vi "VI-Center XControl Property FP Value.vi"(0 "VI in":refnum<vi>, 2 "Data Type In":variant, 11 "error in (no error)":errorcluster) -> (4 "VI out":refnum<vi>, 15 "error out":errorcluster)   [LabVIEW 2015]
uses:
  <vilib>/Utility/traverseref.llb/TRef TravTarget.ctl
panel:
  in  "height":i16=200
  in  "width":i16=200
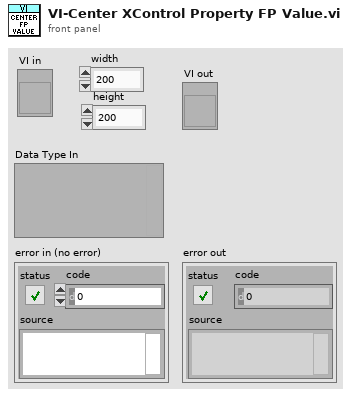
[diagram p1: front panel]
types:
  T1 = typedef "TRef TravTarget.ctl" = enum16{"FP", "BD", "Other"}
  T2 = typedef "LVRectTypeDef.ctl" = cluster{"Left":i16, "Top":i16, "Right":i16, "Bottom":i16}
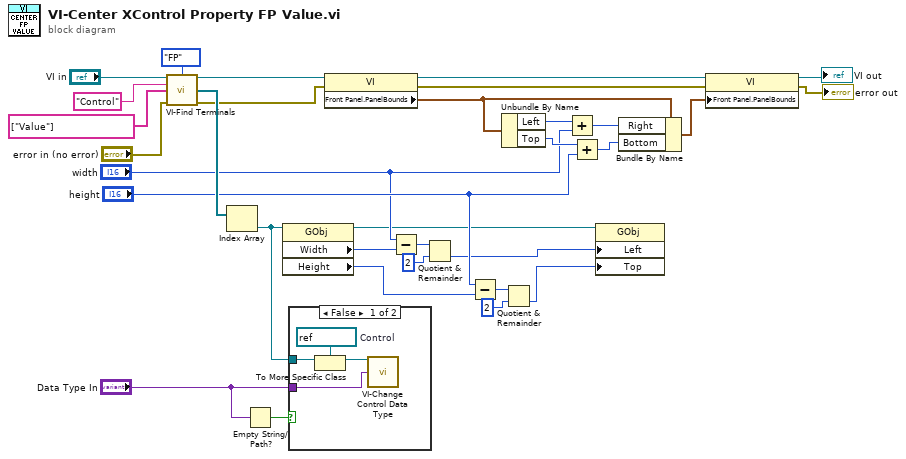
[diagram p0: block diagram]
diagram:
  n1 = call "VI-Find Terminals.vi"("VI in"="VI in", "Traverse Target"=TRef_TravTarget."FP", "Class Name"="Control", "Names"=string[] ["Value"], "error in (no error)"="error in (no error)") -> ("VI out"=w24:refnum<vi>, "Array"=w22:refnum<vi>[], "error out"=w17:errorcluster)  [unwired: 8 in]
  n2 = Index Array(array=w22) -> (element=w3:refnum<vi>)  [unwired: 1 in]
  n3 = Empty String/Path?(string/path="Data Type In") -> (empty?=w1:bool)
  n4 = property class="GObj"(reference=w3) -> (reference out=w5:refnum<vi>, "Width"=w6:u32, "Height"=w7:u32)  [unwired: 1 in, 1 out]
  n5 = case shown="False" w1 {
    tunnel: w3 -> [w34 _]
    tunnel: "Data Type In" -> [w33 _]
    frame False {
      w35 = refnum<vi> refnum  # Control
      n6 = To More Specific Class(target class=w35, reference=w34) -> (specific class reference=w36:refnum<vi>)  [unwired: 1 in, 1 out]
      n7 = call "VI-Change Control Data Type.vi"("Control in"=w36, "Data Type"=w33) -> ()  [unwired: 13 in, 1 out]
    }
    frame True {
    }
  }
  n8 = property class="VI"(reference=w24, error in=w17) -> (reference out=w25:refnum<vi>, error out=w26:errorcluster, "Front Panel.PanelBounds"=w27:T2)
  n9 = Subtract(x="width", y=w6) -> (x-y=w12:u32)
  n10 = Quotient & Remainder(x=w12, y=u32 2) -> (floor(x/y)=w10:u32)  [unwired: 1 out]
  n11 = Subtract(x="height", y=w7) -> (x-y=w9:u32)
  n12 = Unbundle By Name(w27) -> ("Left"=w28:i16, "Top"=w30:i16)
  n13 = Quotient & Remainder(x=w9, y=u32 2) -> (floor(x/y)=w4:u32)  [unwired: 1 out]
  n14 = Add(x=w28, y="width") -> (x+y=w29:i16)
  n15 = Add(x=w30, y="height") -> (x+y=w31:i16)
  n16 = property class="GObj"(reference=w5, "Left"=w10, "Top"=w4) -> ()  [unwired: 1 in, 2 out]
  n17 = Bundle By Name(cluster=w27, "Right"=w29, "Bottom"=w31) -> (w32:T2)
  n18 = property class="VI"(reference=w25, error in=w26, "Front Panel.PanelBounds"=w32) -> (reference out=→"VI out":refnum<vi>, error out=→"error out":errorcluster)
